vi "REPORT.Main others.vi"(7 "file name test":string, 8 "Vasic":i32, 9 "Test IN":T1={"Config HW"={"VISA Rigol DP832"="", "Config Rigol DP832"=[{"Channel"=0, "V Limit"=5.5, "I Limit"=0.5, "V Out"=5.0}, {"Channel"=1, "V Limit"=5.5, "I Limit"=0.8, "V Out"=5.0}, {"Channel"=2, "V Limit"=5.5, "I Limit"=0.2, "V Out"=0.0}], "CTA Test#"="CTA013 A", "FT_Handle"=0, "Espera acceso FT"=10, "VISA Tek MDO3104"="Rigol_DP832", "VISA Key 81160A"="Rigol_DP832"}, "Config Test"=[{"Vasic"=2.8, "Global Reset"=FALSE, "Test Register?"=FALSE, "Test ADC?"=FALSE, "Test ADC"={"Repeats ADC"=100, "Max Desviation"=0.1}, "Limits ADC"={"Low"=[1.9, 1.3, 0.65, 0.0, 1.6, 1.4, 1.4, 0.9, 2.1, 0.85, 1.9], "High"=[2.1, 1.5, 0.85, 0.1, 1.4, 1.2, 1.2, 0.7, 1.9, 0.65, 1.7]}, "Test Max PN Min NP?"=FALSE, "Limits Max PN Min NP"={"Max P Upper"=2.177000045776367, "Min P Upper"=1.474, "Max N Upper"=1.475, "Min N Upper"=0.818, "Max P Lower"=1.888, "Min P Lower "=1.321, "Max N Lower"=1.322, "Min N Lower"=0.73}, "Test Rate Scan?"=FALSE, "Vin Rate Scan"=[], "Limits Rate Scan"={"High"=[0.15, 0.242, 0.331, 0.425, 0.512, 0.6, 0.688, 0.774, 0.847, 0.91], "Low"=[0.021, 0.11, 0.189, 0.27, 0.347, 0.421, 0.487, 0.551, 0.601, 0.635]}, "Test Rate Scan Adders?"=FALSE, "Vin Rate Adders"=[], "Limits Rate Scan adders"={"High"=[], "Low"=[]}, "Test offset analog?"=FALSE, "Lim Offset Analog"={"Max Analog"=0.05, "Min Analog"=-0.05}, "Test offset digital?"=FALSE, "Lim offset Dig"={"Max Dig"=0.05}, "Vasic real f.a."=2.8, "IBIAS"=FALSE, "VALUE IBIAS"=63}, {"Vasic"=2.8, "Global Reset"=FALSE, "Test Register?"=FALSE, "Test ADC?"=FALSE, "Test ADC"={"Repeats ADC"=100, "Max Desviation"=0.1}, "Limits ADC"={"Low"=[1.9, 1.3, 0.65, 0.0, 1.6, 1.4, 1.4, 0.9, 2.1, 0.85, 1.9], "High"=[2.1, 1.5, 0.85, 0.1, 1.4, 1.2, 1.2, 0.7, 1.9, 0.65, 1.7]}, "Test Max PN Min NP?"=FALSE, "Limits Max PN Min NP"={"Max P Upper"=2.177000045776367, "Min P Upper"=1.474, "Max N Upper"=1.475, "Min N Upper"=0.818, "Max P Lower"=1.888, "Min P Lower "=1.321, "Max N Lower"=1.322, "Min N Lower"=0.73}, "Test Rate Scan?"=FALSE, "Vin Rate Scan"=[], "Limits Rate Scan"={"High"=[0.15, 0.242, 0.331, 0.425, 0.512, 0.6, 0.688, 0.774, 0.847, 0.91], "Low"=[0.021, 0.11, 0.189, 0.27, 0.347, 0.421, 0.487, 0.551, 0.601, 0.635]}, "Test Rate Scan Adders?"=FALSE, "Vin Rate Adders"=[], "Limits Rate Scan adders"={"High"=[], "Low"=[]}, "Test offset analog?"=FALSE, "Lim Offset Analog"={"Max Analog"=0.05, "Min Analog"=-0.05}, "Test offset digital?"=FALSE, "Lim offset Dig"={"Max Dig"=0.05}, "Vasic real f.a."=2.8, "IBIAS"=FALSE, "VALUE IBIAS"=63}, {"Vasic"=2.8, "Global Reset"=FALSE, "Test Register?"=FALSE, "Test ADC?"=FALSE, "Test ADC"={"Repeats ADC"=100, "Max Desviation"=0.1}, "Limits ADC"={"Low"=[1.9, 1.3, 0.65, 0.0, 1.6, 1.4, 1.4, 0.9, 2.1, 0.85, 1.9], "High"=[2.1, 1.5, 0.85, 0.1, 1.4, 1.2, 1.2, 0.7, 1.9, 0.65, 1.7]}, "Test Max PN Min NP?"=FALSE, "Limits Max PN Min NP"={"Max P Upper"=2.177000045776367, "Min P Upper"=1.474, "Max N Upper"=1.475, "Min N Upper"=0.818, "Max P Lower"=1.888, "Min P Lower "=1.321, "Max N Lower"=1.322, "Min N Lower"=0.73}, "Test Rate Scan?"=FALSE, "Vin Rate Scan"=[], "Limits Rate Scan"={"High"=[0.15, 0.242, 0.331, 0.425, 0.512, 0.6, 0.688, 0.774, 0.847, 0.91], "Low"=[0.021, 0.11, 0.189, 0.27, 0.347, 0.421, 0.487, 0.551, 0.601, 0.635]}, "Test Rate Scan Adders?"=FALSE, "Vin Rate Adders"=[], "Limits Rate Scan adders"={"High"=[], "Low"=[]}, "Test offset analog?"=FALSE, "Lim Offset Analog"={"Max Analog"=0.05, "Min Analog"=-0.05}, "Test offset digital?"=FALSE, "Lim offset Dig"={"Max Dig"=0.05}, "Vasic real f.a."=2.8, "IBIAS"=FALSE, "VALUE IBIAS"=63}, {"Vasic"=2.8, "Global Reset"=FALSE, "Test Register?"=FALSE, "Test ADC?"=FALSE, "Test ADC"={"Repeats ADC"=100, "Max Desviation"=0.1}, "Limits ADC"={"Low"=[1.9, 1.3, 0.65, 0.0, 1.6, 1.4, 1.4, 0.9, 2.1, 0.85, 1.9], "High"=[2.1, 1.5, 0.85, 0.1, 1.4, 1.2, 1.2, 0.7, 1.9, 0.65, 1.7]}, "Test Max PN Min NP?"=FALSE, "Limits Max PN Min NP"={"Max P Upper"=2.177000045776367, "Min P Upper"=1.474, "Max N Upper"=1.475, "Min N Upper"=0.818, "Max P Lower"=1.888, "Min P Lower "=1.321, "Max N Lower"=1.322, "Min N Lower"=0.73}, "Test Rate Scan?"=FALSE, "Vin Rate Scan"=[], "Limits Rate Scan"={"High"=[0.15, 0.242, 0.331, 0.425, 0.512, 0.6, 0.688, 0.774, 0.847, 0.91], "Low"=[0.021, 0.11, 0.189, 0.27, 0.347, 0.421, 0.487, 0.551, 0.601, 0.635]}, "Test Rate Scan Adders?"=FALSE, "Vin Rate Adders"=[], "Limits Rate Scan adders"={"High"=[], "Low"=[]}, "Test offset analog?"=FALSE, "Lim Offset Analog"={"Max Analog"=0.05, "Min Analog"=-0.05}, "Test offset digital?"=FALSE, "Lim offset Dig"={"Max Dig"=0.05}, "Vasic real f.a."=2.8, "IBIAS"=FALSE, "VALUE IBIAS"=63}], "Result"=[], "Execucion Test"={"Vasic Actual"=0}, "Config VGA"={"Theoretical Voltage"=[0.1, 0.2, 0.3, 0.4, 0.5, 0.6, 0.7, 0.8, 0.9, 1.0], "Real Voltage"=[0.10285, 0.20714, 0.29957, 0.40485, 0.49571, 0.60685, 0.69771, 0.80114, 0.89714, 0.99885], "Pulse Width"=57344, "Frecuency Pulse"=1000000.0, "VGA Gain"=[9, 16, 24, 34, 43, 52, 61, 72, 81, 93]}, "Test Info"={"Asic"="", "Operator"="", "Place"="", "Time start"=timestamp(0 s since 1904-01-01), "Time stop"=timestamp(0 s since 1904-01-01)}, "Info machine"={"SO"="", "SO Name"="", "SO Ver"="", "SO Build"="", "CPU"="", "APP"="", "APP YEAR"="", "APP ver"="", "APP User"="", "APP Serail"="", "MAC"=[], "PC NAME"=[], "PC IP"=[], "BIOS MANU"="", "BIOS NAME"="", "BIOS SERIAL"="", "BOARD MANU"="", "BOARD NAME"="", "BOARD SERIAL"="", "Driver Version"="", "Library Version"="", "FPGA Ver"=0, "ID CTA board"=0, "LAST BOOT"="", "LABVIEW Ver"=0}, "Partial Report"="", "CONFIG GEN"=[]} {"CONFIG GEN"."Vasic Theorical" min=1.0 max=1000000.0 step=1.0 format="%#_6pV"; "CONFIG GEN"."Frequency" min=0.001 max=333000000.0 step=1000.0 format="%#_6pHz"; "CONFIG GEN"."Leading Edge Time" min=1e-09 max=1.0 step=1e-10 format="%#_6ps"; "CONFIG GEN"."Trailing Edge Time" min=1e-09 max=1.0 step=1e-10 format="%#_6ps"; "CONFIG GEN"."Delay" min=0.0 max=1.0 step=1e-12 format="%#_6ps"; "CONFIG GEN"."Trigger Level Sync" items=["ECL", "TTL"]; "CONFIG GEN"."Trigger Sync Out" items=["AB"=3, "B"=2, "A"=1, "None"=0]; "CONFIG GEN"."Load" min=1.0 max=1000000.0 step=1.0 format="%#_6p"; "CONFIG GEN"."DC Offset" min=-10.0 max=10.0 step=0.1 format="%#_6pV"; "CONFIG GEN"."Amplitude" min=0.05 max=5.0 step=0.001 format="%#_6pV"; "CONFIG GEN"."Width Time" min=1.5e-09 max=1.0 step=1e-10 format="%#_6ps"; "CONFIG GEN"."Channel" items=["Channel1"=1, "Channel2"=2]; "Config VGA"."Theoretical Voltage" format="%1.4f"; "Config VGA"."VGA Gain" format="%02x"; "Config VGA"."Frecuency Pulse" format="%0_2p"; "Config VGA"."Pulse Width" format="%04x"; "Config VGA"."Real Voltage" format="%1.5f"; "Config Test"."VALUE IBIAS" max=63 step=1; "Config Test"."Vasic real f.a." min=2.8 max=3.8 step=0.01 format="%.2g"; "Config Test"."Limits Rate Scan adders"."Low" format="%1.3f"; "Config Test"."Limits Rate Scan adders"."High" format="%1.3f"; "Config Test"."Limits ADC"."High" format="%1.4f"; "Config Test"."Limits ADC"."Low" format="%1.3f"; "Config Test"."Lim offset Dig"."Max Dig" format="%.3g"; "Config Test"."Lim Offset Analog"."Min Analog" format="%.3g"; "Config Test"."Lim Offset Analog"."Max Analog" format="%.3g"; "Config Test"."Limits Rate Scan"."Low" format="%1.4f"; "Config Test"."Limits Rate Scan"."High" format="%1.3f"; "Config Test"."Limits Max PN Min NP"."Min P Upper" format="%.3g"; "Config Test"."Limits Max PN Min NP"."Min P Lower" format="%.3g"; "Config Test"."Limits Max PN Min NP"."Max N Lower" format="%.3g"; "Config Test"."Limits Max PN Min NP"."Max N Upper" format="%.3g"; "Config Test"."Limits Max PN Min NP"."Min N Lower" format="%.3g"; "Config Test"."Limits Max PN Min NP"."Min N Upper" format="%.3g"; "Config Test"."Limits Max PN Min NP"."Max P Upper" format="%.3g"; "Config Test"."Limits Max PN Min NP"."Max P Lower" format="%.3g"; "Config Test"."Vasic" min=2.8 max=3.8 step=0.01 format="%.2g"; "Config HW"."Config Rigol DP832"."Channel" items=["+30V Channel 1", "+30V Channel 2", "+5V Channel 3"]; "Config HW"."Config Rigol DP832"."V Limit" format="%.1g"; "Config HW"."Config Rigol DP832"."I Limit" format="%.1g"; "Config HW"."Config Rigol DP832"."V Out" format="%.1g"; "Result"."Test Registros"."Read W/R" format="%04x"; "Result"."Test Registros"."Pattern W/R" format="%04x"; "Result"."Test Registros"."Read Default" format="%04x"; "Result"."Test Registros"."Pattern Default" format="%04x"}, 10 "CSV IN":string) -> (3 "CSV OUT":string)   [LabVIEW 2019]
uses:
  Test.ctl
  TEST.TEST CONFIG HW.ctl
  Rigol DP832/DP832_Control Channels.ctl
  TEST.TEST CONFIG TEST MATRIZ.ctl
  TEST.TEST CONFIG TEST.ctl
  TEST.TEST RESULT.ctl
  test_result fvasic.ctl
  TEST.TEST EXECUTION TEST.ctl
  TEST.TEST CONFIG VGA.ctl
  TEST.TEST TEST INFO.ctl
  TEST.TEST INFO PC.ctl
  GenPulse_configurar.ctl
  Global cuenta erroes.vi
panel:
  # "Modo 2\nModo 3\nModo 4\nModo 2\nModo 3\nModo 4"
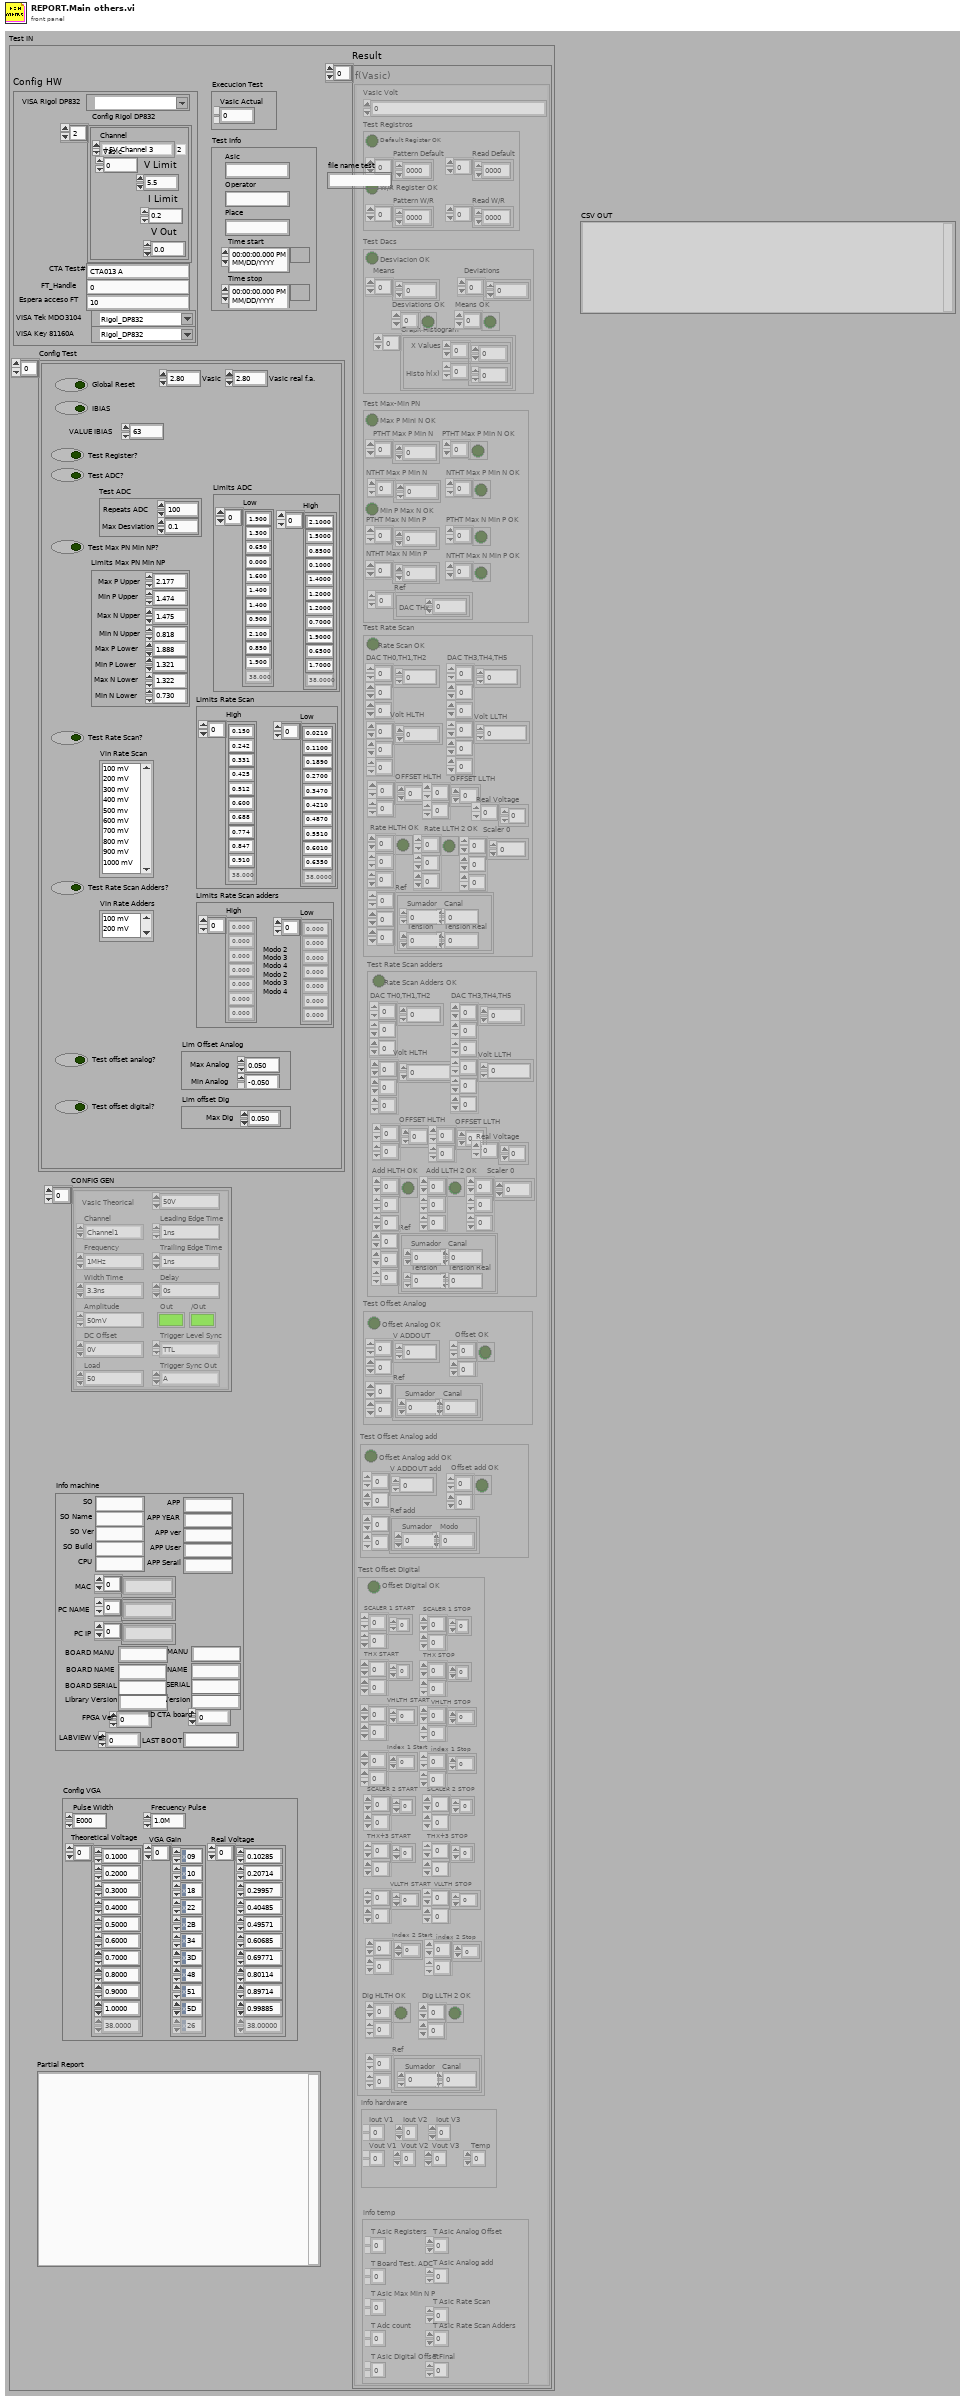
[diagram p1: front panel]
types:
  T1 = typedef "Test.ctl" = cluster{"Config HW":T2, "Config Test":T4, "Result":T6, "Execucion Test":T8, "Config VGA":T9, "Test Info":T10, "Info machine":T11, "Partial Report":string, "CONFIG GEN":T12[]}
  T2 = typedef "TEST.TEST CONFIG HW.ctl" = cluster{"VISA Rigol DP832":refnum<visa-resource-name>, "Config Rigol DP832":cluster{"Channel":T3, "V Limit":dbl, "I Limit":dbl, "V Out":dbl}[], "CTA Test#":string, "FT_Handle":u32, "Espera acceso FT":u32, "VISA Tek MDO3104":refnum<visa-resource-name>, "VISA Key 81160A":refnum<visa-resource-name>}
  T3 = typedef "DP832_Control Channels.ctl" = i32
  T4 = typedef "TEST.TEST CONFIG TEST MATRIZ.ctl" = T5[]
  T5 = typedef "TEST.TEST CONFIG TEST.ctl" = cluster{"Vasic":dbl, "Global Reset":bool, "Test Register?":bool, "Test ADC?":bool, "Test ADC":cluster{"Repeats ADC":i32, "Max Desviation":dbl}, "Limits ADC":cluster{"Low":dbl[], "High":dbl[]}, "Test Max PN Min NP?":bool, "Limits Max PN Min NP":cluster{"Max P Upper":dbl, "Min P Upper":dbl, "Max N Upper":dbl, "Min N Upper":dbl, "Max P Lower":dbl, "Min P Lower ":dbl, "Max N Lower":dbl, "Min N Lower":dbl}, "Test Rate Scan?":bool, "Vin Rate Scan":i32[], "Limits Rate Scan":cluster{"High":dbl[], "Low":dbl[]}, "Test Rate Scan Adders?":bool, "Vin Rate Adders":i32[], "Limits Rate Scan adders":cluster{"High":dbl[], "Low":dbl[]}, "Test offset analog?":bool, "Lim Offset Analog":cluster{"Max Analog":dbl, "Min Analog":dbl}, "Test offset digital?":bool, "Lim offset Dig":cluster{"Max Dig":dbl}, "Vasic real f.a.":dbl, "IBIAS":bool, "VALUE IBIAS":u8}
  T6 = typedef "TEST.TEST RESULT.ctl" = T7[]
  T7 = typedef "test_result fvasic.ctl" = cluster{"Vasic Volt":i32, "Test Registros":cluster{"Default Register OK":bool, "Pattern Default":u16[], "Read Default":u16[], "W/R Register OK":bool, "Pattern W/R":u16[], "Read W/R":u16[]}, "Test Dacs":cluster{"Desviacion OK":bool, "Means":dbl[], "Deviations":dbl[], "Desviations OK":bool[], "Means OK":bool[], "Graph Histogram":cluster{"X Values":dbl[], "Histo h(x)":i32[]}[]}, "Test Max-Min PN":cluster{"Max P Mini N OK":bool, "PTHT Max P Min N":dbl[], "PTHT Max P Min N OK":bool[], "NTHT Max P Min N":dbl[], "NTHT Max P Min N OK":bool[], "Min P Max N OK":bool, "PTHT Max N Min P":dbl[], "PTHT Max N Min P OK":bool[], "NTHT Max N Min P":dbl[], "NTHT Max N Min P OK":bool[], "Ref":cluster{"DAC THx":u8}[]}, "Test Rate Scan":cluster{"Rate Scan OK":bool, "DAC TH0,TH1,TH2":u16[][][], "Volt HLTH":dbl[][][], "Rate HLTH OK":bool[][][], "DAC TH3,TH4,TH5":u16[][][], "Volt LLTH":dbl[][][], "Rate LLTH 2 OK":bool[][][], "Scaler 0":u16[][][], "Ref":cluster{"Sumador":u8, "Canal":u8, "Tension":u8, "Tension Real":dbl}[][][], "OFFSET HLTH":dbl[][], "OFFSET LLTH":dbl[][], "Real Voltage":dbl[]}, "Test Rate Scan adders":cluster{"Rate Scan Adders OK":bool, "DAC TH0,TH1,TH2":u16[][][], "Volt HLTH":dbl[][][], "Add HLTH OK":bool[][][], "DAC TH3,TH4,TH5":u16[][][], "Volt LLTH":dbl[][][], "Add LLTH 2 OK":bool[][][], "Scaler 0":u16[][][], "Ref":cluster{"Sumador":u8, "Canal":u8, "Tension":u8, "Tension Real":dbl}[][][], "OFFSET HLTH":dbl[][], "OFFSET LLTH":dbl[][], "Real Voltage":dbl[]}, "Test Offset Analog":cluster{"Offset Analog OK":bool, "V ADDOUT":dbl[][], "Offset OK":bool[][], "Ref":cluster{"Sumador":u8, "Canal":u8}[][]}, "Test Offset Digital":cluster{"Offset Digital OK":bool, "SCALER 1 START":u16[][], "SCALER 1 STOP":u16[][], "THX START":u16[][], "THX STOP":u16[][], "VHLTH START":dbl[][], "VHLTH STOP":dbl[][], "Index 1 Start":i32[][], "index 1 Stop":i32[][], "SCALER 2 START":u16[][], "SCALER 2 STOP":u16[][], "THX+3 START":u16[][], "THX+3 STOP":u16[][], "VLLTH START":dbl[][], "VLLTH STOP":dbl[][], "Index 2 Start":i32[][], "index 2 Stop":i32[][], "Dig HLTH OK":bool[][], "Dig LLTH 2 OK":bool[][], "Ref":cluster{"Sumador":u8, "Canal":u8}[][]}, "info hardware":cluster{"Iout V1":dbl, "Iout V2":dbl, "Iout V3":dbl, "Vout V1":dbl, "Vout V2":dbl, "Vout V3":dbl, "Temp":dbl}, "Test Offset Analog add":cluster{"Offset Analog add OK":bool, "V ADDOUT add":dbl[][], "Offset add OK":bool[][], "Ref add":cluster{"Sumador":u8, "Modo":u8}[][]}, "info temp":cluster{"T Asic Registers":dbl, "T Board Test. ADC":dbl, "T Asic Max Min N P":dbl, "T Adc count":dbl, "T Asic Digital Offset":dbl, "T Asic Analog Offset":dbl, "T Asic Analog add":dbl, "T Asic Rate Scan":dbl, "T Asic Rate Scan Adders":dbl, "T Final":dbl}}
  T8 = typedef "TEST.TEST EXECUTION TEST.ctl" = cluster{"Vasic Actual":i32}
  T9 = typedef "TEST.TEST CONFIG VGA.ctl" = cluster{"Theoretical Voltage":dbl[], "Real Voltage":dbl[], "Pulse Width":u16, "Frecuency Pulse":dbl, "VGA Gain":u8[]}
  T10 = typedef "TEST.TEST TEST INFO.ctl" = cluster{"Asic":string, "Operator":string, "Place":string, "Time start":timestamp, "Time stop":timestamp}
  T11 = typedef "TEST.TEST INFO PC.ctl" = cluster{"SO":string, "SO Name":string, "SO Ver":string, "SO Build":string, "CPU":string, "APP":string, "APP YEAR":string, "APP ver":string, "APP User":string, "APP Serail":string, "MAC":string[], "PC NAME":string[], "PC IP":string[], "BIOS MANU":string, "BIOS NAME":string, "BIOS SERIAL":string, "BOARD MANU":string, "BOARD NAME":string, "BOARD SERIAL":string, "Driver Version":string, "Library Version":string, "FPGA Ver":u8, "ID CTA board":u64, "LAST BOOT":string, "LABVIEW Ver":u32}
  T12 = typedef "GenPulse_configurar.ctl" = cluster{"Channel":u16, "Frequency":dbl, "Width Time":dbl, "Amplitude":dbl, "DC Offset":dbl, "Load":dbl, "Leading Edge Time":dbl, "Trailing Edge Time":dbl, "Delay":dbl, "Out":bool, "/Out":bool, "Trigger Level Sync":u16, "Trigger Sync Out":u16, "Vasic Theorical":dbl}
  T13 = typedef "global erroes cluster.ctl" = cluster{"Errores FPGA":i32, "Errores Asic":i32, "Errores ADC adq":i32, "Errores ADC Asic":i32}
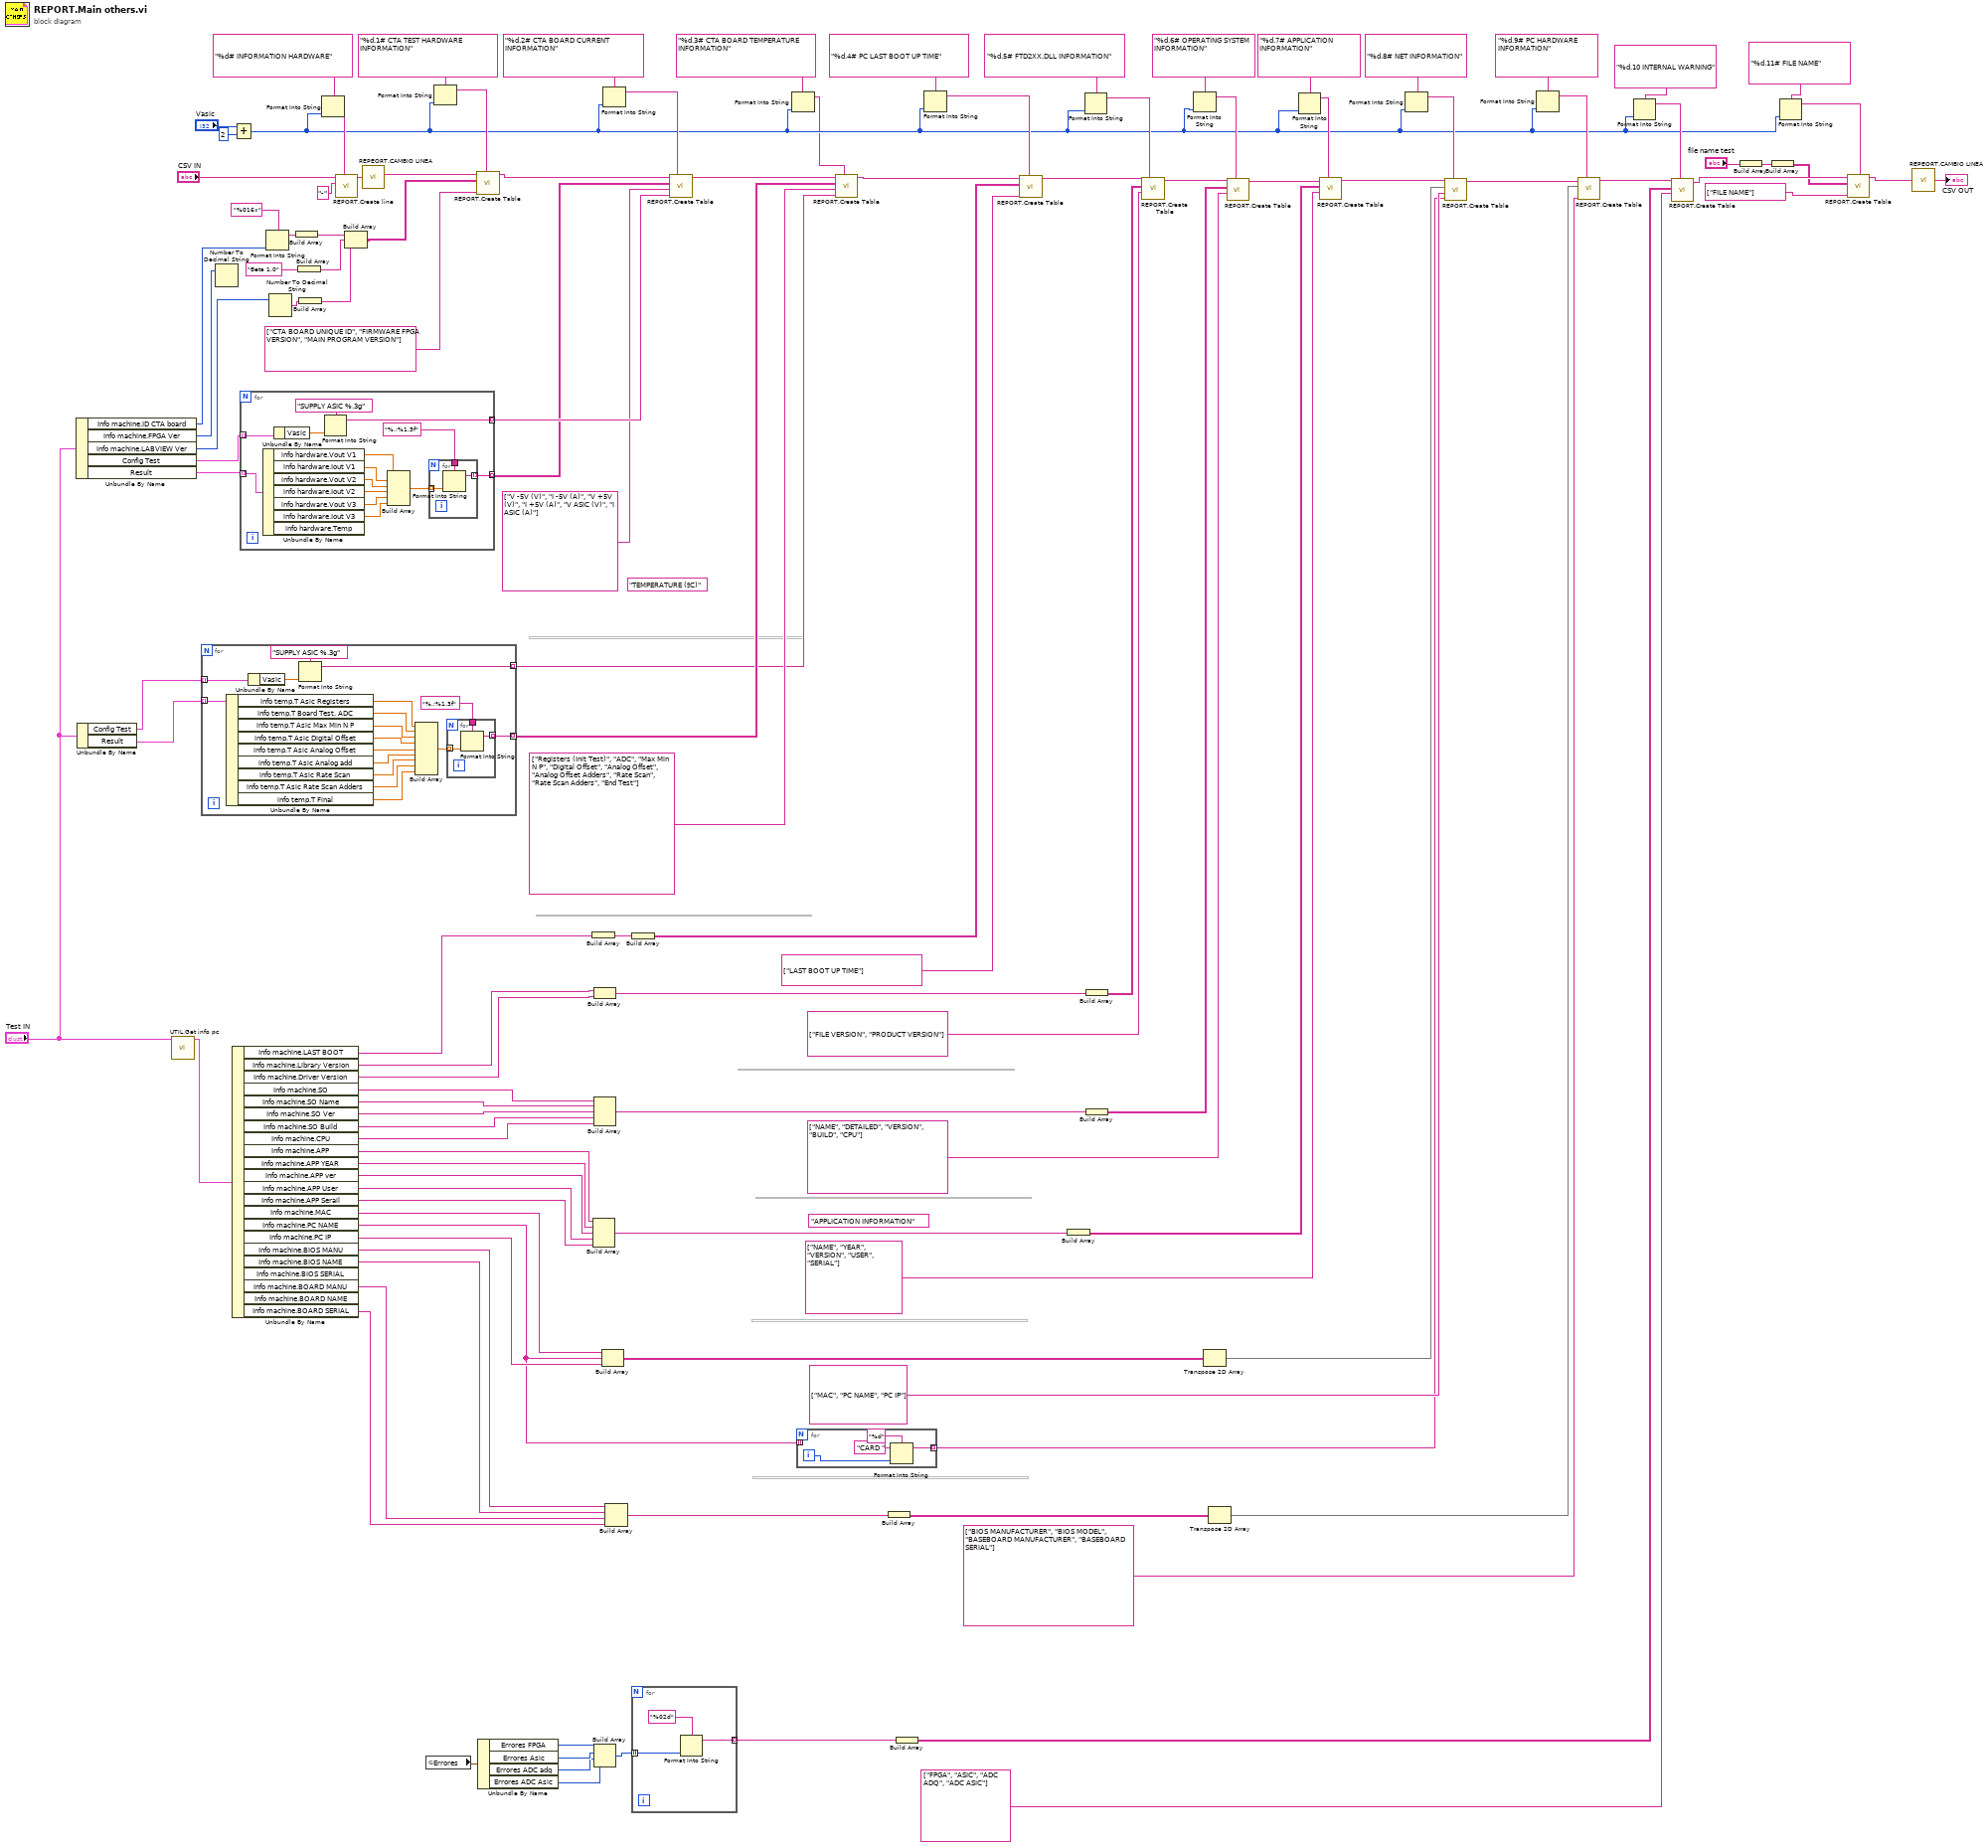
[diagram p0: block diagram]
diagram:
  (unwired) "TEMPERATURE (ºC)"
  (unwired) "APPLICATION INFORMATION"
  n1 = Unbundle By Name("Test IN") -> ("Info machine.ID CTA board"=w21:u64, "Info machine.FPGA Ver"=w20:u8, "Info machine.LABVIEW Ver"=w19:u32, "Config Test"=w58:T4, "Result"=w59:T6)
  n2 = Unbundle By Name("Test IN") -> ("Config Test"=w3:T4, "Result"=w8:T6)
  n3 = call "UTIL.Get info pc.vi"("Test IN"="Test IN") -> ("Test OUT"=w80:T1)  [unwired: 13 in, 1 out]
  n4 = for {
    tunnel: w8 -> [w137] mode=indexing
    tunnel: [w125] -> w5 mode=indexing
    tunnel: w3 -> [w122] mode=indexing
    tunnel: [w121] -> w2 mode=indexing
    n5 = Unbundle By Name(w137) -> ("info temp.T Asic Registers"=w136:dbl, "info temp.T Board Test. ADC"=w135:dbl, "info temp.T Asic Max Min N P"=w134:dbl, "info temp.T Asic Digital Offset"=w133:dbl, "info temp.T Asic Analog Offset"=w132:dbl, "info temp.T Asic Analog add"=w131:dbl, "info temp.T Asic Rate Scan"=w130:dbl, "info temp.T Asic Rate Scan Adders"=w129:dbl, "info temp.T Final"=w128:dbl)
    n6 = Unbundle By Name(w122) -> ("Vasic"=w123:dbl)
    n7 = Format Into String(format string="SUPPLY ASIC %.3g", w123) -> (resulting string=w121:string)  [unwired: 2 in, 1 out]
    n8 = Build Array(w136, w135, w134, w133, w132, w131, w130, w129, w128) -> (w127:dbl[])
    n9 = for {
      tunnel: w127 -> [w140] mode=indexing
      tunnel: "%,;%1.3f" ("format string") -> [w139]
      tunnel: [w138] -> w125 mode=indexing
      n10 = Format Into String(format string=w139, w140) -> (resulting string=w138:string)  [unwired: 2 in, 1 out]
    }
  }
  n11 = Number To Decimal String(number=w20) -> ()  [unwired: 1 in, 1 out]
  n12 = Add(x="Vasic", y=2) -> (x+y=w11:i32)
  n13 = Unbundle By Name(w80) -> ("Info machine.LAST BOOT"=w34:string, "Info machine.Library Version"=w85:string, "Info machine.Driver Version"=w84:string, "Info machine.SO"=w120:string, "Info machine.SO Name"=w119:string, "Info machine.SO Ver"=w118:string, "Info machine.SO Build"=w117:string, "Info machine.CPU"=w116:string, "Info machine.APP"=w115:string, "Info machine.APP YEAR"=w114:string, "Info machine.APP ver"=w113:string, "Info machine.APP User"=w112:string, "Info machine.APP Serail"=w111:string, "Info machine.MAC"=w106:string[], "Info machine.PC NAME"=w99:string[], "Info machine.PC IP"=w105:string[], "Info machine.BIOS MANU"=w101:string, "Info machine.BIOS NAME"=w98:string, "Info machine.BOARD MANU"=w90:string, "Info machine.BOARD SERIAL"=w89:string)  [unwired: 2 out]
  n14 = for {
    tunnel: w59 -> [w154] mode=indexing
    tunnel: w58 -> [w153] mode=indexing
    tunnel: [w151] -> w57 mode=indexing
    tunnel: [w143] -> w55 mode=indexing
    n15 = Unbundle By Name(w154) -> ("info hardware.Vout V1"=w149:dbl, "info hardware.Iout V1"=w148:dbl, "info hardware.Vout V2"=w147:dbl, "info hardware.Iout V2"=w146:dbl, "info hardware.Vout V3"=w145:dbl, "info hardware.Iout V3"=w144:dbl)  [unwired: 1 out]
    n16 = Unbundle By Name(w153) -> ("Vasic"=w152:dbl)
    n17 = Format Into String(format string="SUPPLY ASIC %.3g", w152) -> (resulting string=w151:string)  [unwired: 2 in, 1 out]
    n18 = Build Array(w149, w148, w147, w146, w145, w144) -> (w142:dbl[])
    n19 = for {
      tunnel: w142 -> [w157] mode=indexing
      tunnel: "%,;%1.3f" ("format string") -> [w156]
      tunnel: [w155] -> w143 mode=indexing
      n20 = Format Into String(format string=w156, w157) -> (resulting string=w155:string)  [unwired: 2 in, 1 out]
    }
  }
  n21 = Format Into String(format string="%016x", w21) -> (resulting string=w16:string)  [unwired: 2 in, 1 out]
  n22 = Number To Decimal String(number=w19) -> (decimal integer string=w17:string)  [unwired: 1 in]
  n23 = Build Array(w16) -> (w15:string[])
  n24 = Build Array("Beta 1.0" ("Date")) -> (w14:string[])
  n25 = Build Array(w17) -> (w13:string[])
  n26 = Format Into String(format string="%d# INFORMATION HARDWARE" ("Secction"), w11) -> (resulting string=w74:string)  [unwired: 2 in, 1 out]
  n27 = call "REPORT.Create line.vi"("Secction"=w74, "Char"="-", "Text In"="CSV IN") -> ("Text Out"=w76:string)  [unwired: 8 in]
  n28 = Build Array(w15, w14, w13) -> (w18:string[][])
  n29 = call "REPEORT.CAMBIO LINEA.vi"("Text Out"=w76) -> ("String"=w53:string)  [unwired: 8 in]
  n30 = global read "Global cuenta erroes.vi" "Errores"() -> (w45:T13)
  n31 = Format Into String(format string="%d.1# CTA TEST HARDWARE INFORMATION" ("Secction"), w11) -> (resulting string=w51:string)  [unwired: 2 in, 1 out]
  n32 = call "REPORT.Create Table.vi"("Secction"=w51, "Row Headers"=string[] ["CTA BOARD UNIQUE ID", "FIRMWARE FPGA VERSION", "MAIN PROGRAM VERSION"], "Text 2d"=w18, "Text In"=w53) -> ("Text Out"=w52:string)  [unwired: 4 in, 1 out]
  n33 = Unbundle By Name(w45) -> ("Errores FPGA"=w44:i32, "Errores Asic"=w43:i32, "Errores ADC adq"=w42:i32, "Errores ADC Asic"=w41:i32)
  n34 = Build Array(w34) -> (w32:string[])
  n35 = Build Array(w115, w114, w113, w112, w111) -> (w109:string[])
  n36 = Build Array(w85, w84) -> (w86:string[])
  n37 = Build Array(w120, w119, w118, w117, w116) -> (w110:string[])
  n38 = Build Array(w44, w43, w42, w41) -> (w40:i32[])
  n39 = Build Array(w106, w99, w105) -> (w107:string[][])
  n40 = Format Into String(format string="%d.2# CTA BOARD CURRENT INFORMATION" ("Secction"), w11) -> (resulting string=w60:string)  [unwired: 2 in, 1 out]
  n41 = Build Array(w101, w98, w90, w89) -> (w102:string[])
  n42 = Build Array(w32) -> (w31:string[][])
  n43 = for {
    tunnel: w40 -> [w159] mode=indexing
    tunnel: [w158] -> w39 mode=indexing
    n44 = Format Into String(format string="%02d", w159) -> (resulting string=w158:string)  [unwired: 2 in, 1 out]
  }
  n45 = call "REPORT.Create Table.vi"("Secction"=w60, "Row Headers"=w57, "Column Headers"=string[] ["V -5V (V)", "I -5V (A)", "V +5V (V)", "I +5V (A)", "V ASIC (V)", "I ASIC (A)"], "Text 2d"=w55, "Text In"=w52) -> ("Text Out"=w7:string)  [unwired: 3 in, 1 out]
  n46 = Format Into String(format string="%d.3# CTA BOARD TEMPERATURE INFORMATION" ("Secction"), w11) -> (resulting string=w10:string)  [unwired: 2 in, 1 out]
  n47 = for {
    tunnel: w99 -> [_] mode=indexing
    tunnel: [w161] -> w94 mode=indexing
    i -> [w162]
    n48 = Format Into String(format string="%d", initial string="CARD ", w162) -> (resulting string=w161:string)  [unwired: 1 in, 1 out]
  }
  n49 = call "REPORT.Create Table.vi"("Secction"=w10, "Row Headers"=w2, "Column Headers"=string[] ["Registers (Init Test)", "ADC", "Max Min N P", "Digital Offset", "Analog Offset", "Analog Offset Adders", "Rate Scan", "Rate Scan Adders", "End Test"], "Text 2d"=w5, "Text In"=w7) -> ("Text Out"=w6:string)  [unwired: 3 in, 1 out]
  n50 = Build Array(w102) -> (w97:string[][])
  n51 = Build Array(w39) -> (w38:string[][])
  n52 = Format Into String(format string="%d.4# PC LAST BOOT UP TIME" ("Secction"), w11) -> (resulting string=w33:string)  [unwired: 2 in, 1 out]
  n53 = call "REPORT.Create Table.vi"("Secction"=w33, "Row Headers"=string[] ["LAST BOOT UP TIME"], "Text 2d"=w31, "Text In"=w6) -> ("Text Out"=w35:string)  [unwired: 4 in, 1 out]
  n54 = Build Array(w109) -> (w96:string[][])
  n55 = Format Into String(format string="%d.5# FTD2XX.DLL INFORMATION" ("Secction"), w11) -> (resulting string=w70:string)  [unwired: 2 in, 1 out]
  n56 = Build Array(w86) -> (w83:string[][])
  n57 = Build Array(w110) -> (w91:string[][])
  n58 = call "REPORT.Create Table.vi"("Secction"=w70, "Column Headers"=string[] ["FILE VERSION", "PRODUCT VERSION"], "Text 2d"=w83, "Text In"=w35) -> ("Text Out"=w81:string)  [unwired: 4 in, 1 out]
  n59 = Format Into String(format string="%d.6# OPERATING SYSTEM INFORMATION" ("Secction"), w11) -> (resulting string=w68:string)  [unwired: 2 in, 1 out]
  n60 = Transpose 2D Array(2D array=w107) -> (transposed array=w104:string[][])
  n61 = Transpose 2D Array(2D array=w97) -> (transposed array=w87:string[][])
  n62 = call "REPORT.Create Table.vi"("Secction"=w68, "Column Headers"=string[] ["NAME", "DETAILED", "VERSION", "BUILD", "CPU"], "Text 2d"=w91, "Text In"=w81) -> ("Text Out"=w108:string)  [unwired: 4 in, 1 out]
  n63 = Format Into String(format string="%d.7# APPLICATION INFORMATION" ("Secction"), w11) -> (resulting string=w66:string)  [unwired: 2 in, 1 out]
  n64 = call "REPORT.Create Table.vi"("Secction"=w66, "Column Headers"=string[] ["NAME", "YEAR", "VERSION", "USER", "SERIAL"], "Text 2d"=w96, "Text In"=w108) -> ("Text Out"=w103:string)  [unwired: 4 in, 1 out]
  n65 = Format Into String(format string="%d.8# NET INFORMATION" ("Secction"), w11) -> (resulting string=w64:string)  [unwired: 2 in, 1 out]
  n66 = call "REPORT.Create Table.vi"("Secction"=w64, "Row Headers"=w94, "Column Headers"=string[] ["MAC", "PC NAME", "PC IP"], "Text 2d"=w104, "Text In"=w103) -> ("Text Out"=w100:string)  [unwired: 3 in, 1 out]
  n67 = Format Into String(format string="%d.9# PC HARDWARE INFORMATION" ("Secction"), w11) -> (resulting string=w62:string)  [unwired: 2 in, 1 out]
  n68 = call "REPORT.Create Table.vi"("Secction"=w62, "Row Headers"=string[] ["BIOS MANUFACTURER", "BIOS MODEL", "BASEBOARD MANUFACTURER", "BASEBOARD SERIAL"], "Text 2d"=w87, "Text In"=w100) -> ("Text Out"=w48:string)  [unwired: 4 in, 1 out]
  n69 = Format Into String(format string="%d.10 INTERNAL WARNING" ("Secction"), w11) -> (resulting string=w47:string)  [unwired: 2 in, 1 out]
  n70 = call "REPORT.Create Table.vi"("Secction"=w47, "Column Headers"=string[] ["FPGA", "ASIC", "ADC ADQ", "ADC ASIC"], "Text 2d"=w38, "Text In"=w48) -> ("Text Out"=w28:string)  [unwired: 4 in, 1 out]
  n71 = Build Array("file name test") -> (w26:string[])
  n72 = Build Array(w26) -> (w24:string[][])
  n73 = Format Into String(format string="%d.11# FILE NAME" ("Secction"), w11) -> (resulting string=w23:string)  [unwired: 2 in, 1 out]
  n74 = call "REPORT.Create Table.vi"("Secction"=w23, "Row Headers"=string[] ["FILE NAME"], "Text 2d"=w24, "Text In"=w28) -> ("Text Out"=w27:string)  [unwired: 4 in, 1 out]
  n75 = call "REPEORT.CAMBIO LINEA.vi"("Text Out"=w27) -> ("String"=→"CSV OUT":string)  [unwired: 8 in]
